vi "processPressureString.vi"(8 "error in (no error)":errorcluster, 10 "stringRead":string, 11 "ILC in":refnum<class "ILC.lvclass">) -> (0 "error out":errorcluster, 3 "ILC out":refnum<class "ILC.lvclass">)   [LabVIEW 2015, in "ILCCommon.lvlib" / "ILC.lvclass"]
uses:
  <userlib>/Common/ILC/ILC/ILC.lvclass
  <userlib>/Common/ILC/ILC/ILC.lvclass/ILC.ctl
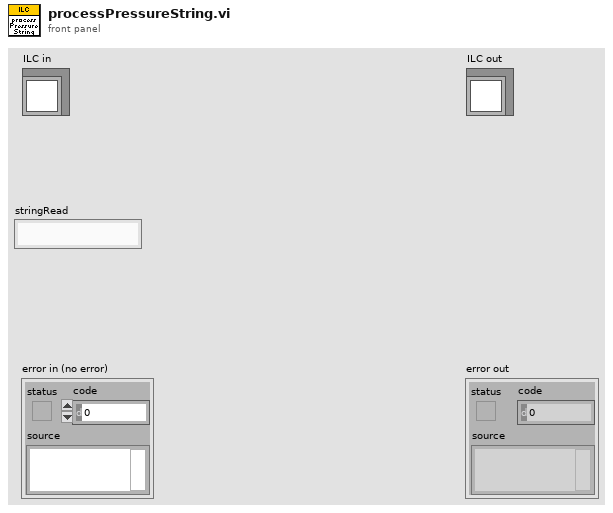
[diagram p1: front panel]
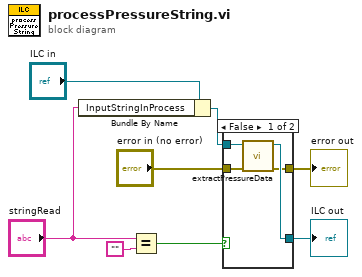
[diagram p0: block diagram]
diagram:
  n1 = Bundle By Name(cluster="ILC in", "InputStringInProcess"="stringRead") -> (w6:refnum<class "ILC.lvclass">)
  n2 = Equal?(x="stringRead", y="") -> (x = y?=w1:bool)
  n3 = case shown="False" w1 {
    tunnel: "error in (no error)" -> [w12 w14]
    tunnel: w6 -> [w11 w13]
    tunnel: [w9 w14] -> w5
    tunnel: [w10 w13] -> w4
    frame False {
      n4 = call <userlib>:"extractPressureData.vi"("error in (no error)"=w12, "ILC in"=w11) -> ("error out"=w9:errorcluster, "ILC out"=w10:refnum<class "ILC.lvclass">)  [unwired: 8 in]
    }
    frame True {
    }
  }
  "error out" <- w5
  "ILC out" <- w4
